vi "PXI-Set AO Config.vi"(0 "AO Channels":i32[](array[numeric]), 1 "Vmax":dbl=10.0, 2 "Vmin":dbl=-10.0, 5 "Sampling Rate (Hz)":dbl, 7 "Buffer Size":i32, 9 "Terminal configuration":i32(ring)=-1 items=["Default"=-1, "RSE"=10083, "Differential"=10106, "Pseudodifferential"=12529], 11 "error in (no error)":errorcluster, 12 "Regenerate":bool=TRUE) -> (15 "error out":errorcluster)   [LabVIEW 2020]
uses:
  Type Defs/Channel Struct.ctl
  DAQ Engine VIs/PXI Globals.vi
panel:
  in  "dummy chan struct":T1={"Channel name"="AI1", "Vmax"=10.0, "Vmin"=10.0, "Rate"=204800.0, "Terminal configuration"=-1, "Physical Channel"="", "Regenerate"=FALSE} {"Terminal configuration" items=["Default"=-1, "RSE"=10083, "Differential"=10106, "Pseudodifferential"=12529]}
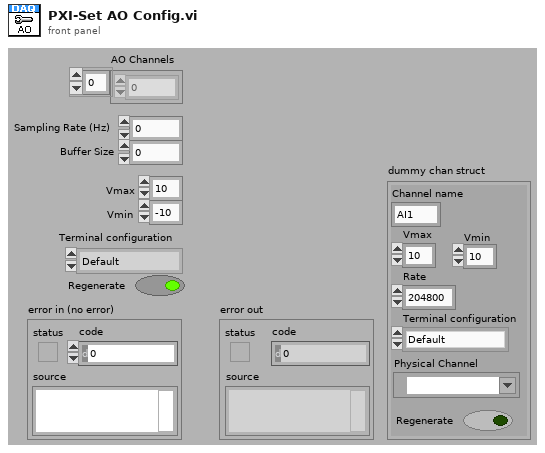
[diagram p1: front panel]
types:
  T1 = typedef "Channel Struct.ctl" = cluster{"Channel name":string, "Vmax":dbl, "Vmin":dbl, "Rate":dbl, "Terminal configuration":i32, "Physical Channel":tag, "Regenerate":bool}
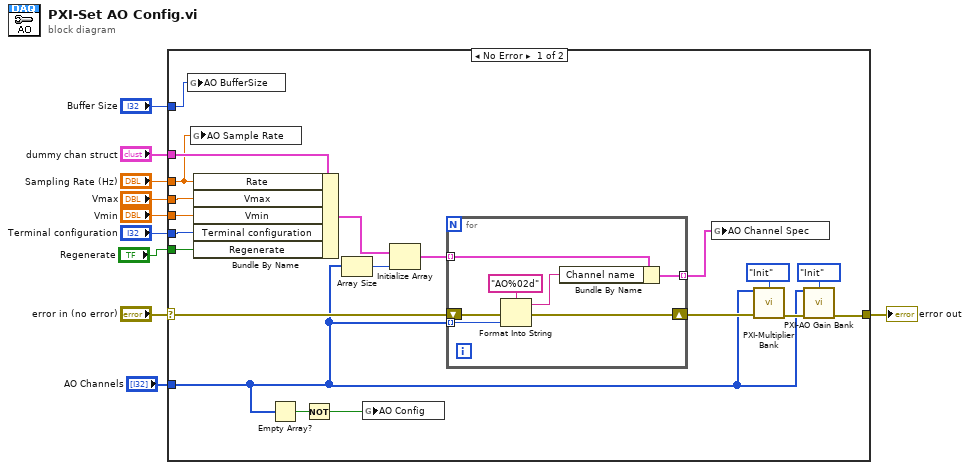
[diagram p0: block diagram]
diagram:
  n1 = case shown="No Error" "error in (no error)" {
    selector: "error in (no error)" -> [w24 w38]
    tunnel: "Terminal configuration" -> [w30 _]
    tunnel: "Vmin" -> [w29 _]
    tunnel: "Vmax" -> [w28 _]
    tunnel: "Sampling Rate (Hz)" -> [w21 _]
    tunnel: "dummy chan struct" -> [w27 _]
    tunnel: "AO Channels" -> [w14 _]
    tunnel: "Buffer Size" -> [w13 _]
    tunnel: [w11 w38] -> w2
    tunnel: "Regenerate" -> [w22 _]
    frame No Error {
      n2 = global write "PXI Globals.vi" "AO BufferSize"(w13) -> ()
      n3 = global write "PXI Globals.vi" "AO Sample Rate"(w21) -> ()
      n4 = Bundle By Name(cluster=w27, "Rate"=w21, "Vmax"=w28, "Vmin"=w29, "Terminal configuration"=w30, "Regenerate"=w22) -> (w26:T1)
      n5 = Empty Array?(array=w14) -> (empty?=w16:bool)
      n6 = Not(x=w16) -> (.not. x?=w15:bool)
      n7 = Array Size(array=w14) -> (size(s)=w12:i32)
      n8 = global write "PXI Globals.vi" "AO Config"(w15) -> ()
      n9 = Initialize Array(w26, w12) -> (w25:T1[])
      n10 = for {
        tunnel: w14 -> [w36] mode=indexing
        tunnel: w25 -> [w35] mode=indexing
        tunnel: [w33] -> w23 mode=indexing
        shift-right: [w31] -> w20
        shift-left: w24 -> [w32]
        n11 = Format Into String(format string="AO%02d", error in=w32, w36) -> (resulting string=w34:string, error out=w31:errorcluster)  [unwired: 1 in]
        n12 = Bundle By Name(cluster=w35, "Channel name"=w34) -> (w33:T1)
      }
      n13 = global write "PXI Globals.vi" "AO Channel Spec"(w23) -> ()
      n14 = call "PXI-Multiplier Bank.vi"("AO Channels"=w14, "Action"=enum16{"Init", "Write", "Read"}."Init", "error in (no error)"=w20) -> ("error out"=w19:errorcluster)  [unwired: 10 in, 2 out]
      n15 = call "PXI-AO Gain Bank.vi"("AO Channels"=w14, "Action"=enum16{"Init", "Write", "Read"}."Init", "error in (no error)"=w19) -> ("error out"=w11:errorcluster)  [unwired: 7 in, 5 out]
    }
    frame Error {
    }
  }
  "error out" <- w2
